vi "Dashboard Main.vi"() -> ()   [LabVIEW 2015]
uses:
  <vilib>/Utility/miscctls.llb/LVRowAndColumnTypeDef.ctl
  <vilib>/event_ctls.llb/eventvkey.ctl
  <vilib>/Rock Robotics/WPI/Dashboard/WPI_DashboardLogging Global.vi
  <vilib>/Rock Robotics/Network Tables/NT Read Numeric Array.vi
  <vilib>/Rock Robotics/Network Tables/NT Read Boolean.vi
  <vilib>/Rock Robotics/Network Tables/NT Write Boolean.vi
  <vilib>/Rock Robotics/Network Tables/NT Write Boolean Array.vi
  <vilib>/Rock Robotics/Network Tables/NT Write Numeric Array.vi
  <vilib>/Utility/config.llb/Write Key (String).vi
  <vilib>/Utility/config.llb/Write Key (I32).vi
  <vilib>/Utility/config.llb/NI_LVConfig.lvlib
panel:
  in  "TCP":refnum<k5>
  in  "Rec Mode":enum32{"Stop", "Record", "Playback"}(radio)
  in  "Vision":u16(ring)=1 items=["Camera Off", "USB Camera SW", "USB Camera HW", "IP Camera"]
  out "Camera IP":string
  out "Image Message":string="Timeout in Camera Communications"
  in  "Dashboard Tab":T1(tab)
  in  "Select Auto":string(combo)
  out "NT Connection":bool
  in  "Camera Settings":T2={"Frame Rate"=30, "Compression"=30, "Size"=1} {"Frame Rate" scale=1.0..30.0; "Size" items=["640x480", "320x240", "160x120"]}
  out "MotorChart R":cluster{"Numeric":dbl, "Numeric":dbl}(graph)
  out "MotorChart L":T3(graph)
  out "MotorSliders R":cluster{"MotorSlide1":dbl, "MotorSlide2":dbl} {"MotorSlide2" scale=-1.0..1.0 scale format="%#_2e"; "MotorSlide1" scale=-1.0..1.0 scale format="%#_2e"}
  out "MotorSliders L":T4 {"MotorSlide4 2" scale=0.0..14.0 scale format="%#_2e"; "MotorSlide2" scale=-1.0..1.0 scale format="%#_2e"; "MotorSlide1" scale=-1.0..1.0 scale format="%#_2e"}
  out "Gyro":dbl(knob) scale=0.0..360.0
  out "JS1 Z":dbl(slide) scale=-1.0..1.0 scale format="%#_2e"
  out "JS1 Graph":cluster{"X":dbl, "Y":dbl}[](graph)
  out "JS1 Buttons":T5
  out "JS2 Z":dbl(slide) scale=-1.0..1.0 scale format="%#_2e"
  out "JS2 Graph":cluster{"X":dbl, "Y":dbl}[](graph)
  out "JS2 Buttons":T5
  out "Mode":T6(ring)=enum."Auto Disabled"
  in  "DB Camera Config":bool
  out "fps":dbl format="%#.1g"
  out "Mbps":dbl format="%#.1g"
  out "Mbps LED":bool
  in  "DB/String 9":string
  in  "DB/String 8":string
  in  "DB/String 7":string
  in  "DB/String 6":string
  in  "DB/String 5":string
  in  "DB/String 4":string
  in  "DB/String 3":string
  in  "DB/String 2":string
  in  "DB/String 1":string
  in  "DB/String 0":string
  in  "DB/Slider 0":dbl(slide) scale=0.0..5.0
  in  "DB/Slider 1":dbl(slide) scale=0.0..5.0
  in  "DB/Slider 2":dbl(slide) scale=0.0..5.0
  in  "DB/Slider 3":dbl(slide) scale=0.0..5.0
  out "DB/LED 3":bool
  out "DB/LED 2":bool
  out "DB/LED 1":bool
  out "DB/LED 0":bool
  in  "DB/Button 3":bool
  in  "DB/Button 2":bool
  in  "DB/Button 1":bool
  in  "DB/Button 0":bool caption="New Name"
  in  "Rampart":bool
  in  "CL":dbl
  in  "Exposure Percentage":dbl
  in  "Brightness":dbl
  in  "Blue":cluster{"Low":dbl, "High":dbl}={"Low"=100.0, "High"=200.0}
  in  "Green":cluster{"Low":dbl, "High":dbl}={"Low"=100.0, "High"=230.0}
  in  "Red":cluster{"Low":dbl, "High":dbl}={"Low"=0.0, "High"=100.0}
  in  "Taking A Shot":bool
  in  "Position 4":bool
  in  "Position 3":bool
  in  "Position 2":bool
  in  "Position 1":bool
  out "Robot Aligned Straight":bool
  out "Ball In Position":bool
  in  "Test Slider":dbl(slide) scale=0.0..100.0 scale format="%#_3g"
  in  "On/Off":bool caption="Solenoid"
  in  "Test Name":u16(ring) items=["Select the test to run..."]
  in  "Test Tree":string(tree)
  in  "Motor":cluster{"Value":dbl, "Enable":bool} {"Value" scale=-1.0..1.0 scale format="%#_3g"}
  out "Progress":T7 {"Test Progress" scale=0.0..100.0}
  in  "Rev/Fwd":cluster{"Forward":bool, "Reverse":bool}
  in  "Test Ring":u16(ring) items=["Monochrome", "Color"]
  out "Cmd Status":string
  in  "Execute Command":bool
  in  "Command Params":string[][](table)
  in  "Command Selection":i32(listbox)
  in  "CheckList":i32(listbox)
  out "Tree":string(tree)
  out "Camera Image":T8(plugin-control)
  out "Background":bool
  # "Left"
  # "Front"
  # "Right"
  # "Battery"
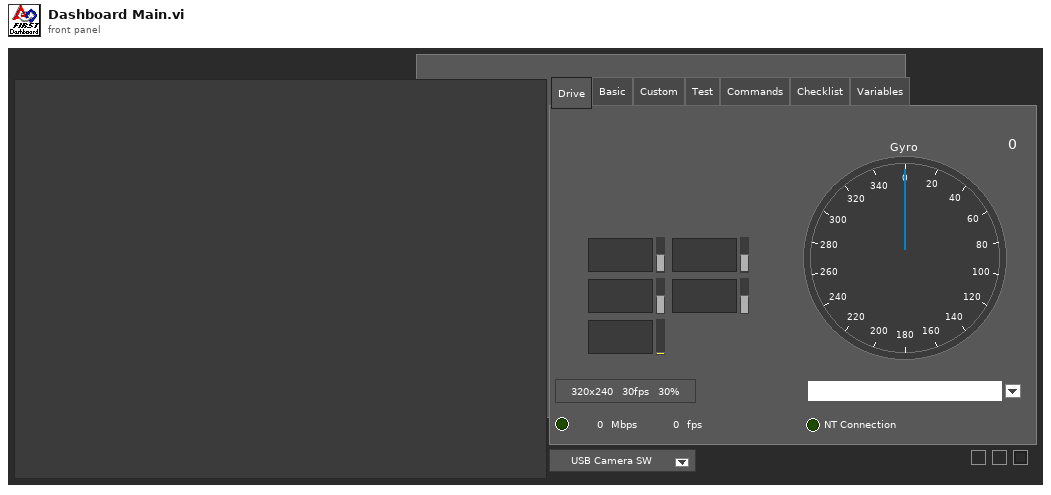
[diagram p1: front panel]
types:
  T1 = enum32{"Drive", "Basic", "Custom", "Test", "Commands", "Checklist", "Variables"}
  T2 = cluster{"Frame Rate":i32, "Compression":i32, "Size":u16}
  T3 = cluster{"Numeric":dbl, "Numeric":dbl, "Battery V":dbl}
  T4 = cluster{"MotorSlide1":dbl, "MotorSlide2":dbl, "MotorSlide4 2":dbl}
  T5 = cluster{bool, bool, bool, bool, bool, bool, bool, bool, bool, bool, bool, bool}
  T6 = enum8{"Tele-Op Disabled", "Tele-Op Enabled", "Auto Disabled", "Auto Enabled", "Test Disabled", "Test Enabled", "Disconnected", "No Code", "E-Stop"}
  T7 = cluster{"Test Progress":u8, "Test Progress Text":string}
  T8 = typedef "IMAQ Image.ctl" = refnum<image>
  T9 = cluster{"IDs":cluster{"RPC field ID":u16, "Unique ID":u16}, "String":string}
  T10 = enum32{"Drive", "Basic", "Custom", "Test", "Checklist", "Variables"}
  T11 = typedef "Image Type" = u32
  T12 = cluster{"Camera Image":refnum<vi>, "Dashboard Tab":refnum<vi>, "Background":refnum<vi>, "Vision":refnum<vi>, "Rec Mode":refnum<vi>, "Test Slider":refnum<vi>, "On/Off ":refnum<vi>, "Test Ring":refnum<vi>, "Rev/Fwd":refnum<vi>, "Test Name":refnum<vi>, "Motor":refnum<vi>, "Progress":refnum<vi>, "CheckList":refnum<vi>, "Tree":refnum<vi>, "Test Tree":refnum<vi>, "Command Params":refnum<vi>, "Command Selection":refnum<vi>, "Execute Command":refnum<vi>, "Cmd Status":refnum<vi>}
  T13 = cluster{"Error Strings":string, "Disable Counts":cluster{u16, u16}, "Rail Faults":cluster{u16, u16, u16}, "Robot IP":string, "DB Mode":u8, "Event Info":cluster{"Name":string, "Type":u8, "Number":u16, "Replay":u8}, "Camera Addr":string}
  T14 = cluster{"Storage":cluster{"Disk Free":u64, "RAM Block":u32, "RAM free":u32}, "CPU Utilization":cluster{"CPU % ISR":sgl, "CPU % Time Crit":sgl, "CPU % Timed Str":sgl, "CPU % High":sgl, "CPU % Above":sgl, "CPU % Normal":sgl, "CPU % Low":sgl}, "CAN":cluster{"% Bus Utilization":sgl, "Bus Off Cnt":u32, "TX_FIFO Full Cnt":u32, "Receive Error Cnt":u8, "Transmit Error Cnt":u8}, "HID":cluster{"HID Outputs":u32, "Rumble Low":u16, "Rumble High":u16}[]}
  T15 = cluster{"Status bits":cluster{"Test Mode":bool, "Autonomous":bool, "Enabled":bool, "Code Start":bool, "Brownout":bool, "Reserved 2":bool, "Reserved 3":bool, "E-Stop":bool}, "Code Trace":cluster{"Disabled":bool, "TeleOp":bool, "Auto":bool, "Test":bool}, "Controller Type":enum16{"unknown", "cRIO", "roboRio"}, "Code?":enum16{"unknown", "noCode", "code"}, "Battery V":dbl}
  T16 = cluster{"Control Bits":cluster{"TestMode":bool, "Autonomous":bool, "Enabled":bool, "FMS Present":bool, bool, bool, bool, "E-Stop":bool}, "Team Station ":u8, "Countdown":sgl, "Joystick Values":cluster{"Axes":dbl[], "Buttons":bool[], "POVs":i16[]}[]}
  T17 = cluster{"Axes":dbl[], "Buttons":bool[], "POVs":i16[]}[]
  T18 = cluster{"Axes":dbl[], "Buttons":bool[], "POVs":i16[]}
  T19 = cluster{"Buttons[0]":bool, "Buttons[1]":bool, "Buttons[2]":bool, "Buttons[3]":bool, "Buttons[4]":bool, "Buttons[5]":bool, "Buttons[6]":bool, "Buttons[7]":bool, "Buttons[8]":bool, "Buttons[9]":bool, "Buttons[10]":bool, "Buttons[11]":bool}
  T20 = typedef "NI_LVConfig.lvlib/Config Data RefNum.ctl" = refnum<k1>
  T21 = cluster{"Operation":enum16{"Update", "Clear"}, "Color Box":u32}[]
  T22 = typedef "eventvkey.ctl" = enum16{"ASCII", "Enter", "Return", "Shift", "Ctrl", "Alt", "Cmd", "Opt", "Caps", "NumLock", "Clear", "Break", "Up", "Down", "Left", "Right", "Insert", "Delete", "Home", "End", "PageUp", "PageDown", "Escape", "Help", "Pause", "ScrollLock", "F1", "F2", "F3", "F4", "F5", "F6", "F7", "F8", "F9", "F10", "F11", "F12", "F13", "F14", "F15", "F16", "F17", "F18", "F19", "F20", "F21", "F22", "F23", "F24", "Play", "VolumeUp", "VolumeDown", "Mute", "Two Byte Char"}
  T23 = cluster{"Image Size":bool, "Image Type":bool, "Pixel Value":bool, "ROI Information":bool, "Zoom Factor":bool}
  T24 = enum8{"Enabled", "Disabled", "Disabled and Grayed Out"}
  T25 = cluster{"Operation":enum16{"Update", "Clear"}, "Color Box":u32}
  T26 = typedef "LVRowAndColumnTypeDef.ctl" = cluster{"Row":i32, "Column":i32}
  T27 = cluster{"Shift":bool, "Ctrl":bool, "Alt":bool, "Cmd":bool, "Opt":bool}
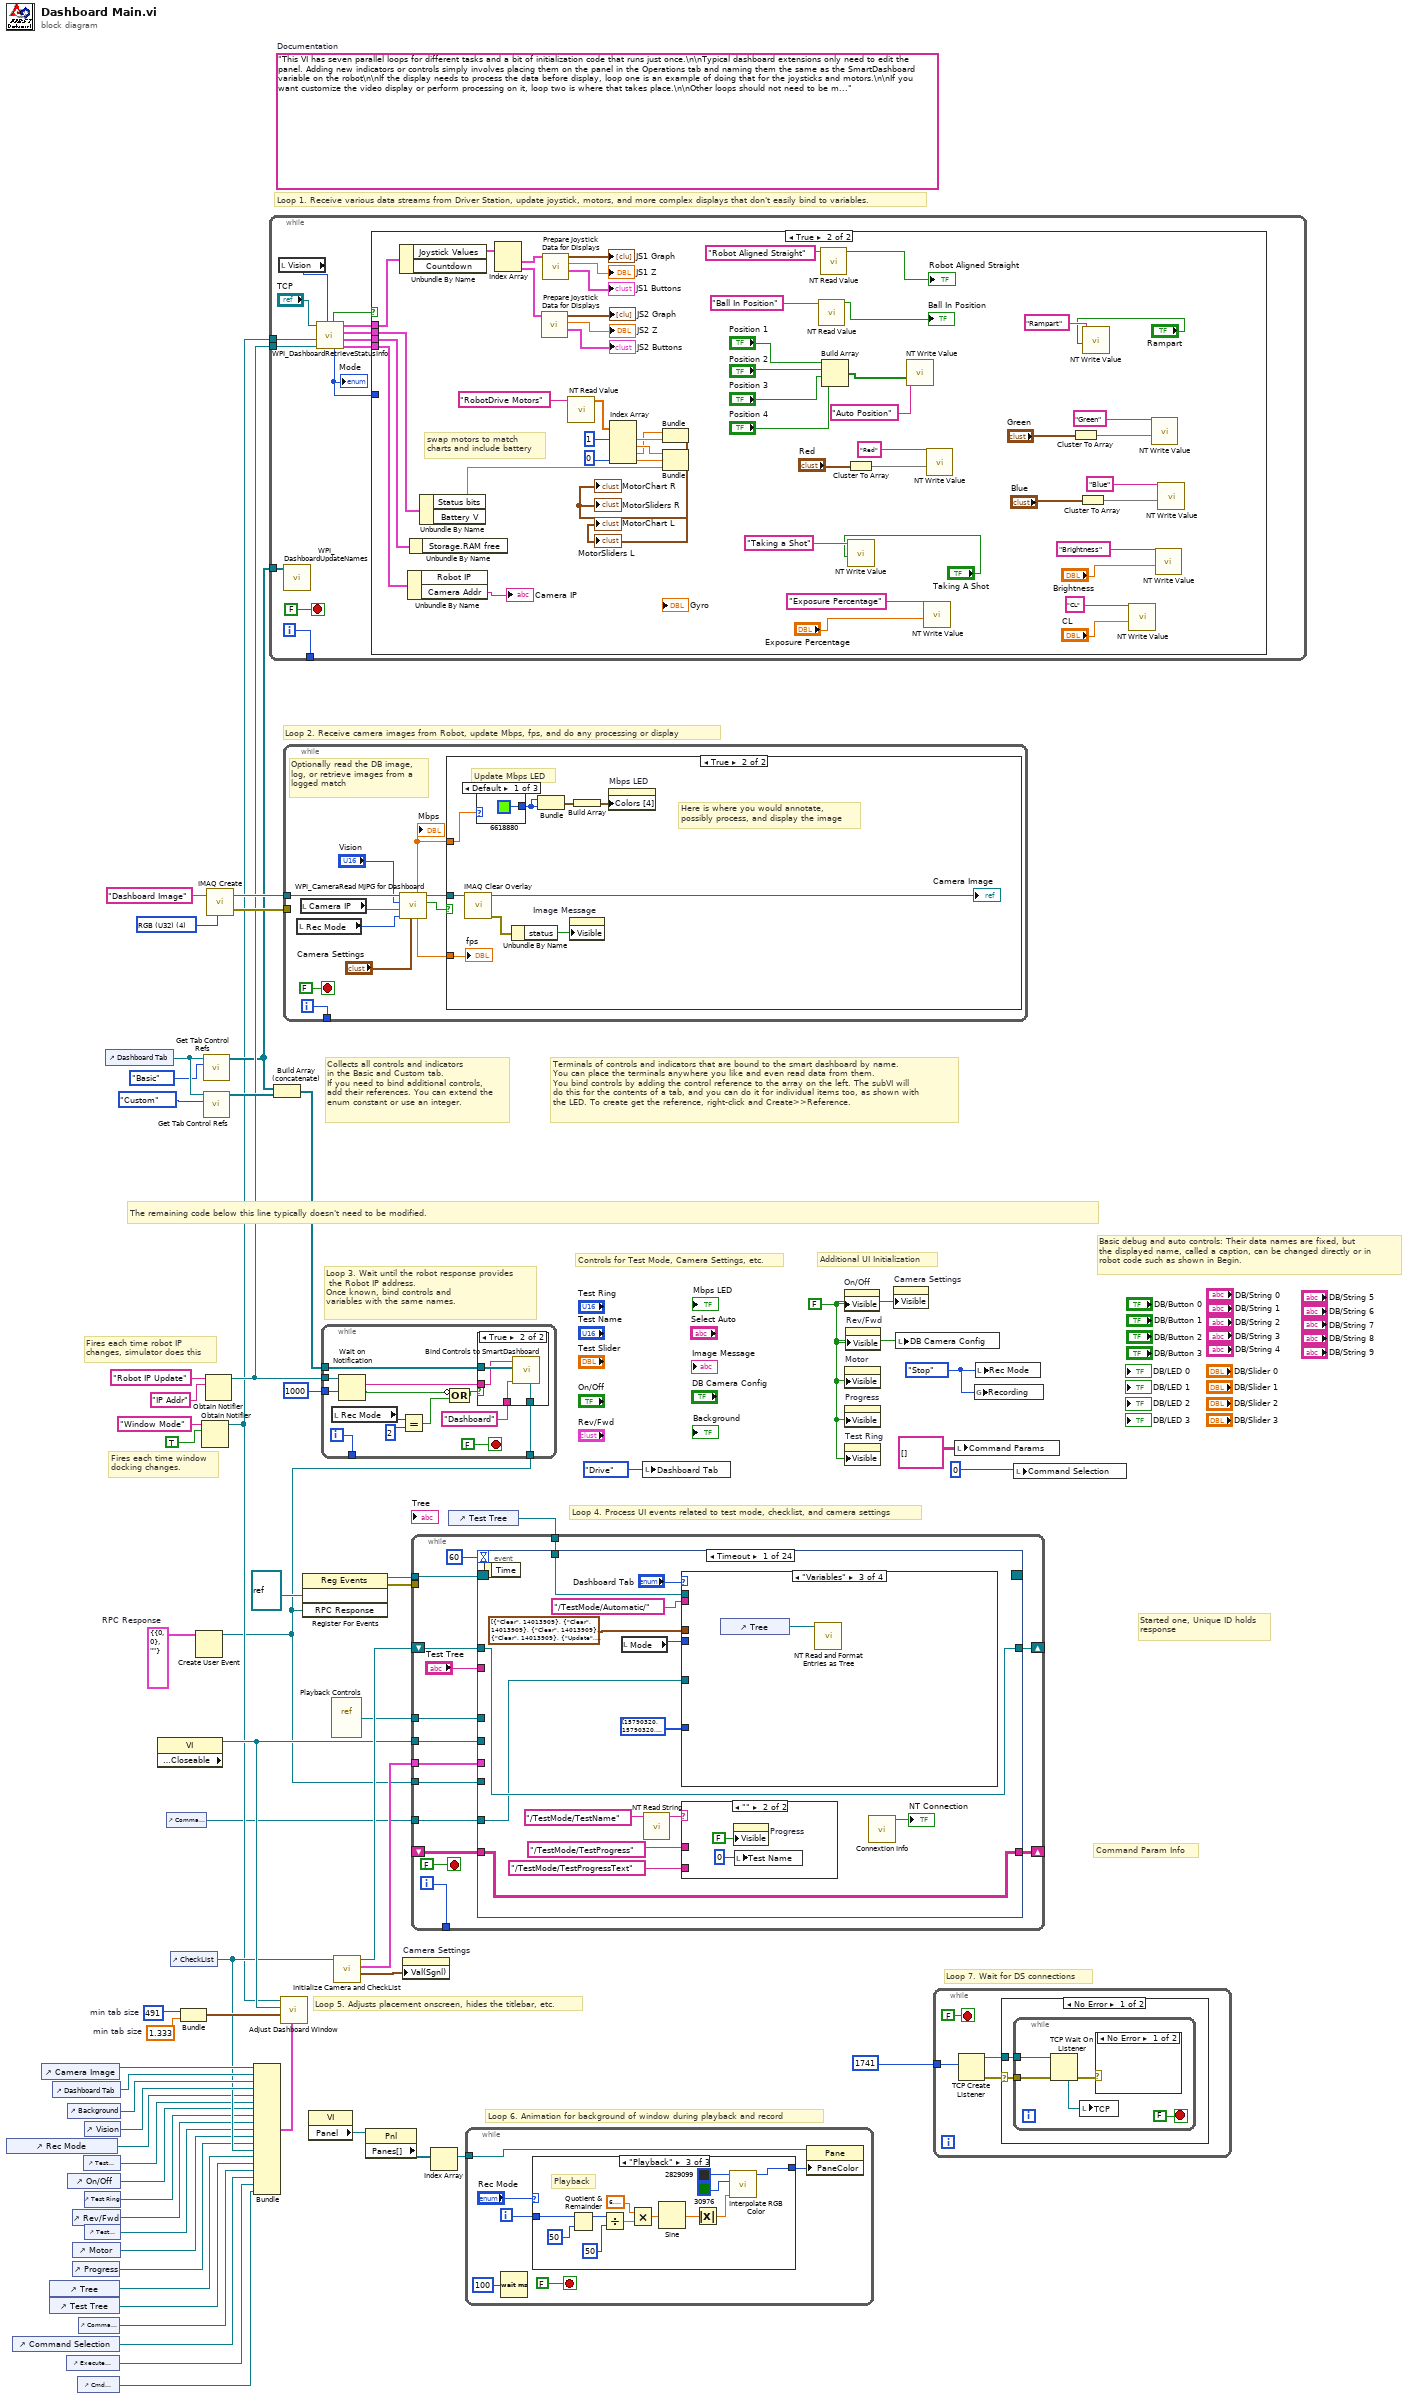
[diagram p0: block diagram]
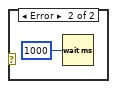
[diagram p2: hidden frame]
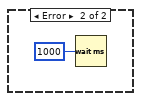
[diagram p3: hidden frame]
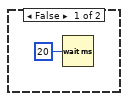
[diagram p4: hidden frame]
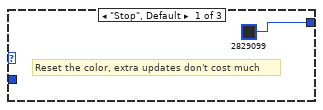
[diagram p5: hidden frame]
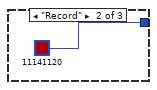
[diagram p6: hidden frame]
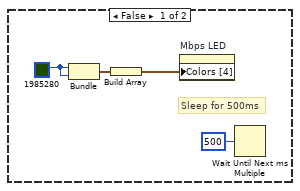
[diagram p8: hidden frame]
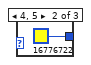
[diagram p9: hidden frame]
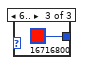
[diagram p10: hidden frame]
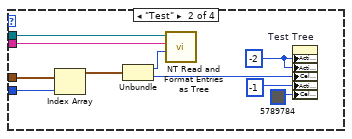
[diagram p12: hidden frame]
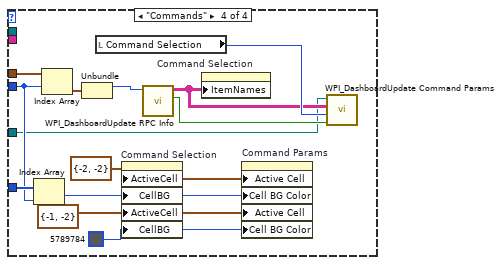
[diagram p13: hidden frame]
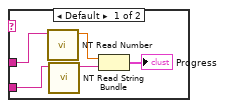
[diagram p14: hidden frame]
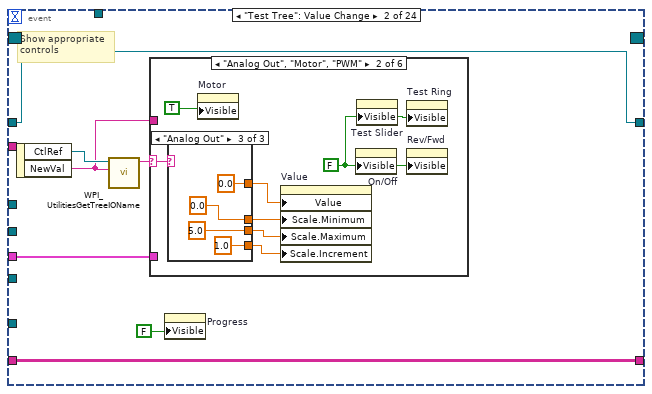
[diagram p15: hidden frame]
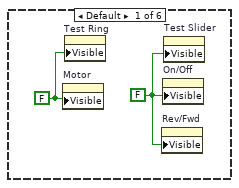
[diagram p16: hidden frame]
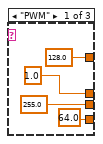
[diagram p17: hidden frame]
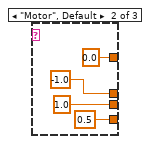
[diagram p18: hidden frame]
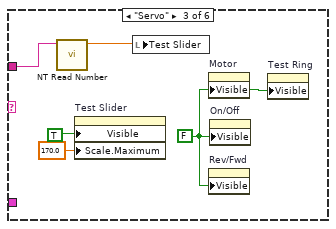
[diagram p19: hidden frame]
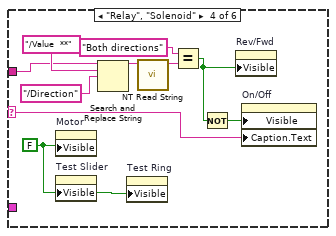
[diagram p20: hidden frame]
diagram:
  w7 = T9 {"IDs"={"RPC field ID"=0, "Unique ID"=0}, "String"=""}  # RPC Response
  w33 = 491  # min tab size
  w32 = 1.333  # min tab size
  w41 = enum32{"Stop", "Record", "Playback"}."Stop" ("Rec Mode")
  w15 = FALSE ("Visible")
  (unwired) "This VI has seven parallel loops for different tasks and a bit of initialization code that runs just once.\n\nTypical dashboard extensions only need to edit the panel. Adding new indicators or controls simply involves placing them on the panel in the Operations tab and naming them the same as the SmartDashboard variable on the robot\n\nIf the display needs to process the data before display, loop one is an example of doing that for the joysticks and motors.\n\nIf you want customize the video display or perform processing on it, loop two is where that takes place.\n\nOther loops should not need to be modified. They are pretty standard, and document the task they perform."  # Documentation
  w61 = T11 4 items=["Grayscale (U8)", "Grayscale (I16)", "Grayscale (SGL)", "Complex (CSG)", "RGB (U32)", "HSL (U32)", "RGB (U64)"] ("Image Type")
  # "Command Param Info"
  # "Started one, Unique ID holds\nresponse"
  # "Loop 7. Wait for DS connections"
  # "Basic debug and auto controls: Their data names are fixed, but\nthe displayed name, called a caption, can be changed directly or in\nrobot code such as shown in Begin."
  # "Controls for Test Mode, Camera Settings, etc."
  # "Additional UI Initialization"
  # "Loop 6. Animation for background of window during playback and record"
  # "Fires each time robot IP\nchanges, simulator does this"
  # "Fires each time window\ndocking changes."
  # "Collects all controls and indicators\nin the Basic and Custom tab.\nIf you need to bind additional controls,\nadd their references. You can extend the\nenum constant or use an integer."
  # "The remaining code below this line typically doesn't need to be modified."
  # "Loop 4. Process UI events related to test mode, checklist, and camera settings"
  # "Terminals of controls and indicators that are bound to the smart dashboard by name.\nYou can place the terminals anywhere you like and even read data from them.\nYou bind controls by adding the control reference to the array on the left. The subVI will\ndo this for the contents of a tab, and you can do it for individual items too, as shown with\nthe LED. To create get the reference, right-click and Create>>Reference."
  # "Loop 3. Wait until the robot response provides\n the Robot IP address.\nOnce known, bind controls and\nvariables with the same names."
  # "Loop 5. Adjusts placement onscreen, hides the titlebar, etc."
  # "Loop 1. Receive various data streams from Driver Station, update joystick, motors, and more complex displays that don't easily bind to variables."
  # "Loop 2. Receive camera images from Robot, update Mbps, fps, and do any processing or display"
  n1 = control-ref of="Rec Mode"() -> (w21:refnum<vi>)
  n2 = control-ref of="Command Selection"() -> (w6:refnum<vi>)
  n3 = control-ref of="Camera Image"() -> (w36:refnum<vi>)
  n4 = control-ref of="Tree"() -> (w25:refnum<vi>)
  n5 = control-ref of="Test Tree"() -> (w24:refnum<vi>)
  n6 = control-ref of="Dashboard Tab"() -> (w35:refnum<vi>)
  n7 = control-ref of="Execute Command"() -> (w8:refnum<vi>)
  n8 = control-ref of="Background"() -> (w30:refnum<vi>)
  n9 = control-ref of="On/Off"() -> (w19:refnum<vi>)
  n10 = control-ref of="Progress"() -> (w16:refnum<vi>)
  n11 = control-ref of="Rev/Fwd"() -> (w17:refnum<vi>)
  n12 = control-ref of="Motor"() -> (w22:refnum<vi>)
  n13 = control-ref of="Cmd Status"() -> (w2:refnum<vi>)
  n14 = control-ref of="Command Params"() -> (w9:refnum<vi>)
  n15 = control-ref of="Test Slider"() -> (w20:refnum<vi>)
  n16 = control-ref of="Vision"() -> (w34:refnum<vi>)
  n17 = control-ref of="Test Ring"() -> (w18:refnum<vi>)
  n18 = control-ref of="Test Name"() -> (w23:refnum<vi>)
  n19 = control-ref of="Dashboard Tab"() -> (w39:refnum<vi>)
  n20 = property class="VI" props=["Front Panel.Closeable"]() -> (reference out=w40:refnum<vi>)  [unwired: 2 in, 2 out]
  n21 = control-ref of="Command Params"() -> (w1:refnum<vi>)
  n22 = control-ref of="CheckList"() -> (w26:refnum<vi>)
  n23 = Bundle("min tab size"=w33, "min tab size"=w32) -> (w31:cluster{"min tab size":i32, "min tab size":dbl})  [unwired: 1 in]
  n24 = Create User Event(user event datatype=w7) -> (user event=w3:refnum<user-event>)  [unwired: 1 in, 1 out]
  n25 = Obtain Notifier(name (unnamed)="Window Mode", notification data type=TRUE) -> (notifier out=w12:refnum<notifier>)  [unwired: 2 in, 2 out]
  n26 = call <vilib>:"Get Tab Control Refs.vi"("Page Index"=T10."Basic" ("Dashboard Tab"), "TabControl in"=w39) -> ("ControlsOnPage"=w13:refnum<vi>[])  [unwired: 9 in]
  n27 = call <vilib>:"Get Tab Control Refs.vi"("Page Index"=T10."Custom" ("Dashboard Tab"), "TabControl in"=w39) -> ("ControlsOnPage"=w38:refnum<vi>[])  [unwired: 9 in]
  n28 = Obtain Notifier(name (unnamed)="Robot IP Update", notification data type="IP Addr" ("name (unnamed)")) -> (notifier out=w14:refnum<notifier>)  [unwired: 2 in, 2 out]
  n29 = call "IMAQ Create"("Image Name"="Dashboard Image", "Image Type"=w61) -> ("New Image"=w59:T8, "error out"=w58:errorcluster)  [unwired: 2 in, 1 out]
  n30 = Bundle("Camera Image"=w36, "Dashboard Tab"=w35, "Background"=w30, "Vision"=w34, "Rec Mode"=w21, "Test Slider"=w20, "On/Off"=w19, "Test Ring"=w18, "Rev/Fwd"=w17, "Test Name"=w23, "Motor"=w22, "Progress"=w16, "CheckList"=w26, "Tree"=w25, "Test Tree"=w24, "Command Params"=w9, "Command Selection"=w6, "Execute Command"=w8, "Cmd Status"=w2) -> (w27:T12)  [unwired: 1 in]
  n31 = while {
    tunnel: [w73] -> _
    tunnel: w14 -> [w67]
    tunnel: w13 -> [w66]
    tunnel: w12 -> [w62]
    i -> [w73]
    stop <- FALSE stop-if-true
    n32 = local read "Vision"() -> (w64:u16)
    n33 = call <vilib>:"WPI_DashboardUpdateNames.vi"("Controls on Tab"=w66) -> ()  [unwired: 11 in]
    n34 = call <vilib>:"WPI_DashboardRetrieveStatusInfo.vi"("Vision"=w64, "Binding Refnum"=w67, "Window Mode Notifier"=w62, "TCP Cnx"="TCP") -> ("Power and Errors"=w68:T13, "Robot Metrics"=w71:T14, "Status Info"=w72:T15, "Control Info"=w69:T16, "Robot Mode"=w65:T6, "Process?"=w70:bool)  [unwired: 2 in]
    "Mode" <- w65
    n35 = case shown="True" w70 {
      tunnel: w72 -> [_ w129]
      tunnel: w71 -> [_ w128]
      tunnel: w69 -> [_ w127]
      tunnel: w68 -> [_ w126]
      tunnel: w65 -> [_ _]
      frame False {
        n36 = Wait (ms)(milliseconds to wait=u32 20) -> ()  [unwired: 1 out]
      }
      frame True {
        # "swap motors to match\ncharts and include battery"
        n37 = Unbundle By Name(w127) -> ("Joystick Values"=w116:T17)  [unwired: 1 out]
        n38 = Unbundle By Name(w126) -> ("Camera Addr"=→"Camera IP":string)  [unwired: 1 out]
        n39 = Unbundle By Name(w128) -> ()  [unwired: 1 out]
        n40 = Unbundle By Name(w129) -> ("Battery V"=w117:dbl)  [unwired: 1 out]
        n41 = Index Array(array=w116) -> (element #1=w115:T18, element #2=w110:T18)  [unwired: 2 in]
        n42 = call "Prepare Joystick Data for Displays.vi"("Joystick Values"=w110) -> ("Buttons"=→"JS2 Buttons":T19, "Z Axis"=→"JS2 Z":dbl, "Cartesian Data"=→"JS2 Graph":cluster{"X axis":dbl, "X axis":dbl}[])  [unwired: 8 in]
        n43 = call "Prepare Joystick Data for Displays.vi"("Joystick Values"=w115) -> ("Buttons"=→"JS1 Buttons":T19, "Z Axis"=→"JS1 Z":dbl, "Cartesian Data"=→"JS1 Graph":cluster{"X axis":dbl, "X axis":dbl}[])  [unwired: 8 in]
        n44 = call-poly <vilib>:"NT Read Value.vi"("Name"="RobotDrive Motors") -> ("Numeric Array"=w105:dbl[])  [unwired: 9 in, 1 out]
        n45 = Index Array(array=w105, index #1=1, index #4=0) -> (element #1=w121:dbl, element #2=w122:dbl, element #3=w120:dbl, element #4=w125:dbl)  [unwired: 2 in]
        n46 = Bundle("Numeric"=w120, "Numeric"=w121) -> (→"MotorChart R" →"MotorSliders R":cluster{"Numeric":dbl, "Numeric":dbl})  [unwired: 1 in]
        n47 = Bundle("Numeric"=w122, "Numeric"=w125, "Battery V"=w117) -> (→"MotorChart L" →"MotorSliders L":T3)  [unwired: 1 in]
        n48 = call-poly <vilib>:"NT Read Value.vi"("Name"="Ball In Position") -> ("Boolean"=→"Ball In Position":bool)  [unwired: 9 in, 1 out]
        n49 = call-poly <vilib>:"NT Read Value.vi"("Name"="Robot Aligned Straight") -> ("Boolean"=→"Robot Aligned Straight":bool)  [unwired: 9 in, 1 out]
        n50 = Build Array("Position 1", "Position 2", "Position 3", "Position 4") -> (w93:bool[])
        n51 = Cluster To Array(cluster="Red") -> (array=w89:dbl[])
        n52 = call-poly <vilib>:"NT Write Value.vi"("Boolean"="Taking A Shot", "Name"="Taking a Shot") -> ()  [unwired: 9 in, 1 out]
        n53 = call-poly <vilib>:"NT Write Value.vi"("Boolean Array"=w93, "Name"="Auto Position") -> ()  [unwired: 9 in, 1 out]
        n54 = call-poly <vilib>:"NT Write Value.vi"("Numeric"="Exposure Percentage", "Name"="Exposure Percentage") -> ()  [unwired: 9 in, 1 out]
        n55 = call-poly <vilib>:"NT Write Value.vi"("Numeric Array"=w89, "Name"="Red") -> ()  [unwired: 9 in, 1 out]
        n56 = Cluster To Array(cluster="Green") -> (array=w88:dbl[])
        n57 = Cluster To Array(cluster="Blue") -> (array=w85:dbl[])
        n58 = call-poly <vilib>:"NT Write Value.vi"("Boolean"="Rampart", "Name"="Rampart") -> ()  [unwired: 9 in, 1 out]
        n59 = call-poly <vilib>:"NT Write Value.vi"("Numeric"="CL", "Name"="CL") -> ()  [unwired: 9 in, 1 out]
        n60 = call-poly <vilib>:"NT Write Value.vi"("Numeric Array"=w88, "Name"="Green") -> ()  [unwired: 9 in, 1 out]
        n61 = call-poly <vilib>:"NT Write Value.vi"("Numeric"="Brightness", "Name"="Brightness") -> ()  [unwired: 9 in, 1 out]
        n62 = call-poly <vilib>:"NT Write Value.vi"("Numeric Array"=w85, "Name"="Blue") -> ()  [unwired: 9 in, 1 out]
      }
    }
  }
  n63 = Build Array (concatenate)(w13, w38) -> (w37:refnum<vi>[])
  n64 = call "Adjust Dashboard Window.vi"("Sizing Refnums"=w27, "Size Constraints"=w31, "VI"=w40, "WIn Mode"=w12) -> ()  [unwired: 8 in]
  n65 = while {
    tunnel: w59 -> [w138]
    tunnel: w58 -> [_]
    tunnel: [w139] -> _
    i -> [w139]
    stop <- FALSE stop-if-true
    # "Optionally read the DB image,\nlog, or retrieve images from a\nlogged match"
    n66 = local read "Rec Mode"() -> (w133:enum32{"Stop", "Record", "Playback"})
    n67 = local read "Camera IP"() -> (w131:string)
    n68 = call <vilib>:"WPI_CameraRead MJPG for Dashboard.vi"("Camera Settings"="Camera Settings", "Rec Mode"=w133, "Camera IP"=w131, "Camera Mode"="Vision", "Refnum in"=w138) -> ("Active"=w136:bool, "Refnum out"=w137:T8, "FPS"=w135:dbl, "Bandwidth (Mbps)"=w130:dbl)  [unwired: 3 in]
    "Mbps" <- w130
    n69 = case shown="True" w136 {
      tunnel: w137 -> [_ w148]
      tunnel: w130 -> [_ w147]
      tunnel: w135 -> [_ w145]
      frame False {
        w141 = u32 1985280 ("Color Box")
        # "Sleep for 500ms"
        n70 = Bundle("Color Box"=w141, "Color Box"=w141) -> (w143:cluster{"Color Box":u32, "Color Box":u32})  [unwired: 1 out]
        n71 = Build Array(w143) -> (w142:cluster{"Color Box":u32, "Color Box":u32}[])
        n72 = property on="Mbps LED" class="Bool (strict)"("Colors [4]"=w142) -> ()  [unwired: 2 in, 2 out]
        n73 = Wait Until Next ms Multiple(millisecond multiple=u32 500) -> ()  [unwired: 1 out]
      }
      frame True {
        # "Here is where you would annotate,\npossibly process, and display the image"
        # "Update Mbps LED"
        n74 = call "IMAQ Clear Overlay"("Image"=w148) -> ("error out"=w152:errorcluster, "Image Out"=→"Camera Image":T8)  [unwired: 2 in, 7 out]
        n75 = case shown="Default" w147 {
          tunnel: [u32 6618880 ("Color Box") u32 16776722 ("Color Box") u32 16716800 ("Color Box")] -> w149
          frame Default {
          }
          frame 4, 5 {
          }
          frame 6.. {
          }
        }
        n76 = Unbundle By Name(w152) -> ("status"=w153:bool)
        n77 = Bundle("Color Box"=w149, "Color Box"=w149) -> (w151:cluster{"Color Box":u32, "Color Box":u32})  [unwired: 1 out]
        n78 = property on="Image Message" class="Str"("Visible"=w153) -> ()  [unwired: 2 in, 2 out]
        n79 = Build Array(w151) -> (w150:cluster{"Color Box":u32, "Color Box":u32}[])
        n80 = property on="Mbps LED" class="Bool (strict)"("Colors [4]"=w150) -> ()  [unwired: 2 in, 2 out]
        "fps" <- w145
      }
    }
  }
  n81 = register-events(refnum<vi> refnum, w3) -> (reference out=w45:refnum<event-registration>, error out=w44:errorcluster)  [unwired: 2 in]
  n82 = property class="VI"() -> ("Panel"=w48:refnum<vi>)  [unwired: 2 in, 2 out]
  n83 = while {
    tunnel: w37 -> [w169]
    tunnel: w14 -> [w167]
    tunnel: [w165] -> _
    tunnel: u32 1000 ("milliseconds to wait") -> [w164]
    tunnel: w3 -> [w157]
    i -> [w165]
    stop <- FALSE stop-if-true
    n84 = local read "Rec Mode"() -> (w160:enum32{"Stop", "Record", "Playback"})
    n85 = Wait on Notification(notifier=w167, timeout in ms (-1)=w164) -> (notification=w166:string, timed out?=w162:bool)  [unwired: 2 in, 2 out]
    n86 = Equal?(x=w160, y=u16 2 ("Rec Mode")) -> (x = y?=w161:bool)
    n87 = Compound Arithmetic op=OR(invert w162, w161) -> (w163:bool)
    n88 = case shown="True" w163 {
      tunnel: w169 -> [_ w173]
      tunnel: w166 -> [_ w172]
      tunnel: "Dashboard" -> [_ w171]
      tunnel: w157 -> [_ w170]
      frame False {
      }
      frame True {
        n89 = call <vilib>:"Bind Controls to SmartDashboard.vi"("RPC ref"=w170, "Client Name"=w171, "Bound Control Refs"=w173, "Server IP Address"=w172) -> ()  [unwired: 8 in]
      }
    }
  }
  n90 = vi-ref "Playback Controls.vi"() -> (w46:refnum<vi>)
  n91 = call "Initialize Camera and CheckList.vi"("ListBox in"=w26) -> ("Cluster"=w52:cluster{"value":i32, "value":i32, "index":i32}, "Array"=w53:cluster{string[]}[], "File Refnum"=w51:T20)  [unwired: 8 in]
  n92 = property class="Pnl"(reference=w48) -> ("Panes[]"=w49:refnum<vi>[])  [unwired: 1 in, 2 out]
  n93 = property on="Camera Settings" class="Clust (strict)"("Val(Sgnl)"=w52) -> ()  [unwired: 2 in, 2 out]
  n94 = Index Array(array=w49) -> (element=w47:refnum<vi>)  [unwired: 1 in]
  n95 = control-ref of="Test Tree"() -> (w50:refnum<vi>)
  n96 = while {
    tunnel: w53 -> [w185]
    shift-right: [w184] -> _
    shift-left: w51 -> [w183]
    tunnel: [w182] -> _
    tunnel: w50 -> [w181]
    tunnel: w46 -> [w180]
    tunnel: w45 -> [w179]
    tunnel: w44 -> [_]
    tunnel: w40 -> [w178]
    tunnel: w3 -> [w177]
    tunnel: w1 -> [w176]
    shift-right: [w175] -> _
    shift-left: _ -> [w174]
    i -> [w182]
    stop <- FALSE stop-if-true
    n97 = event shown="[0] Timeout" {
      selector: w179 -> [_ _ _ _ _ _ _ _ _ _ _ _ _ _ _ _ _ _ _ _ _ _ _ _]
      dyn-events: [_ _ _ _ _ _ _ _ _ _ _ _ _ _ _ _ _ _ w494 _ _ _ _ _] -> _
      timeout: u32 60 ("milliseconds to wait") -> [_ _ _ _ _ _ _ _ _ _ _ _ _ _ _ _ _ _ _ _ _ _ _ _]
      tunnel: w181 -> [w198 _ _ _ _ _ _ _ _ _ _ _ _ _ _ _ _ _ _ _ _ _ _ _]
      tunnel: "Test Tree" -> [_ _ _ _ _ _ _ _ _ _ _ _ _ w457 w466 w469 w474 w483 _ _ _ _ _ _]
      tunnel: w185 -> [_ w236 _ _ _ _ _ _ _ _ _ w419 w450 _ _ _ _ _ _ _ _ _ _ _]
      tunnel: [w195 w235 w339 w345 w355 w359 w365 w377 w385 w391 w404 w418 w443 w456 w464 w468 w473 w482 w496 w512 w514 w522 w533 w538] -> w184
      tunnel: w183 -> [w195 w235 w339 w345 w355 w359 w365 w377 w385 w391 w404 w417 w443 w456 w464 w468 w473 w482 w496 w512 w514 w522 w533 w538]
      tunnel: w180 -> [_ _ _ _ _ _ _ _ _ _ _ _ _ _ _ _ _ _ w497 _ w517 _ _ _]
      tunnel: w178 -> [_ _ _ _ _ _ _ _ _ _ _ _ _ _ _ _ _ _ w492 _ _ _ _ _]
      tunnel: w177 -> [_ _ _ _ _ _ _ _ _ _ _ _ _ _ _ _ _ _ w488 _ _ _ _ _]
      tunnel: w176 -> [w190 _ _ _ _ _ w363 _ _ _ _ _ _ _ _ _ _ _ _ _ _ _ _ _]
      tunnel: [w189 w234 w338 w344 w354 w360 w361 w371 w382 w390 w403 w416 w442 w455 w463 w467 w472 w481 w487 w510 w513 w518 w526 w539] -> w175
      tunnel: w174 -> [w189 w234 w338 w344 w354 w360 w361 _ _ w390 w403 w416 w442 w455 w463 w467 w472 w481 w487 w510 w513 w518 w526 w539]
      event Timeout {
        n98 = event-data() -> ()  [unwired: 1 in, 1 out]
        n99 = local read "Mode"() -> (w192:T6)
        n100 = call <vilib>:"NT Read String.vi"("Name"="/TestMode/TestName") -> ("String"=w201:string)  [unwired: 9 in, 1 out]
        n101 = case shown="\"Variables\"" "Dashboard Tab" {
          tunnel: w198 -> [_ w212 _ _]
          tunnel: "/TestMode/Automatic/" ("Name Pattern") -> [_ w211 _ _]
          tunnel: T21 [{"Operation"=enum."Clear", "Color Box"=14013909}, {"Operation"=enum."Clear", "Color Box"=14013909}, {"Operation"=enum."Clear", "Color Box"=14013909}, {"Operation"=enum."Clear", "Color Box"=14013909}, {"Operation"=enum."Update", "Color Box"=14013909}, {"Operation"=enum."Update", "Color Box"=16777215}, {"Operation"=enum."Clear", "Color Box"=14013909}, {"Operation"=enum."Clear", "Color Box"=14013909}, {"Operation"=enum."Clear", "Color Box"=14013909}] -> [_ w204 _ w221]
          tunnel: w192 -> [_ w203 _ w220]
          tunnel: u32[] [15790320, 15790320, 15790320, 15790320, 16777215, 16777215, 15790320, 15790320, 15790320] -> [_ _ _ w226]
          tunnel: w190 -> [_ _ _ w214]
          frame "Custom", Default {
          }
          frame "Test" {
            w210 = -2 ("Active Item:Row Number")
            n102 = Index Array(array=w204, index=w203) -> (element=w205:T25)
            n103 = Unbundle(w205) -> ("Operation"=w206:enum16{"Update", "Clear"}, "Color Box"=w207:u32)
            n104 = call <vilib>:"NT Read and Format Entries as Tree.vi"("Operation"=w206, "Name Pattern"=w211, "Tree Refnum"=w212) -> ()  [unwired: 7 in, 2 out]
            n105 = property on="Test Tree" class="Tree (strict)"("Active Item Row Number"=w210, "ActiveColNum"=w210, "CellBG"=w207, "Active Item Row Number"=-1 ("Active Item:Row Number"), "CellBG"=u32 5789784 ("Color Box")) -> ()  [unwired: 2 in, 2 out]
          }
          frame "Variables" {
            n106 = control-ref of="Tree"() -> (w213:refnum<vi>)
            n107 = call <vilib>:"NT Read and Format Entries as Tree.vi"("Tree Refnum"=w213) -> ()  [unwired: 9 in, 2 out]
          }
          frame "Commands" {
            w222 = u32 5789784 ("Color Box")
            w223 = T26 {"Row"=-1, "Column"=-2} ("Active Cell:Active Cell")
            w225 = T26 {"Row"=-2, "Column"=-2} ("Active Cell:Active Cell")
            n108 = Index Array(array=w226, index=w220) -> (element=w224:u32)
            n109 = Index Array(array=w221, index=w220) -> (element=w219:T25)
            n110 = Unbundle(w219) -> ("Operation"=w218:enum16{"Update", "Clear"})  [unwired: 1 out]
            n111 = local read "Command Selection"() -> (w217:i32)
            n112 = property on="Command Selection" class="MCListbox (strict)"("ActiveCell"=w225, "CellBG"=w224, "ActiveCell"=w223, "CellBG"=w222) -> ()  [unwired: 2 in, 2 out]
            n113 = call <vilib>:"WPI_DashboardUpdate RPC Info.vi"("Operation"=w218) -> ("update"=w216:bool, "commands"=w215:string[][])  [unwired: 9 in]
            n114 = property on="Command Selection" class="MCListbox (strict)"("ItemNames"=w215) -> ()  [unwired: 2 in, 2 out]
            n115 = property on="Command Params" class="Tbl (strict)"("Active Cell"=w225, "Cell BG Color"=w224, "Active Cell"=w223, "Cell BG Color"=w222) -> ()  [unwired: 2 in, 2 out]
            n116 = call <vilib>:"WPI_DashboardUpdate Command Params.vi"("Update"=w216, "NewVal"=w217, "Commands"=w215, "Param Tbl"=w214) -> ()  [unwired: 7 in, 1 out]
          }
        }
        n117 = case shown="\"\"" w201 {
          tunnel: "/TestMode/TestProgress" ("Name") -> [w228 _]
          tunnel: "/TestMode/TestProgressText" ("Name") -> [w227 _]
          frame Default {
            n118 = call <vilib>:"NT Read Number.vi"("Name"=w228) -> ("Numeric"=w229:dbl)  [unwired: 9 in, 1 out]
            n119 = call <vilib>:"NT Read String.vi"("Name"=w227) -> ("String"=w230:string)  [unwired: 9 in, 1 out]
            n120 = Bundle("Numeric"=w229, "String"=w230) -> (→"Progress":cluster{"Numeric":dbl, "String":string})  [unwired: 1 in]
          }
          frame "" {
            n121 = property on="Progress" class="Clust (strict)"("Visible"=FALSE) -> ()  [unwired: 2 in, 2 out]
            n122 = local write "Test Name"(u16 0) -> ()
          }
        }
        n123 = call <vilib>:"Connextion Info.vi"() -> ("Connected"=→"NT Connection":bool)  [unwired: 10 in, 1 out]
      }
      event "Test Tree": Value Change {
        # "Show appropriate\ncontrols"
        n124 = event-data() -> ("CtlRef"=w239:refnum<vi>, "NewVal"=w237:string)  [unwired: 1 in]
        n125 = call <vilib>:"WPI_UtilitiesGetTreeIOName.vi"("NewVal"=w237, "TreeControl in"=w239) -> ("I/O Name"=w240:string)  [unwired: 9 in]
        n126 = case shown="\"Analog Out\", \"Motor\", \"PWM\"" w240 {
          selector: w240 -> [_ w247 _ w269 w278 _]
          tunnel: w237 -> [_ _ w266 w268 _ w285]
          tunnel: w236 -> [_ _ _ _ _ w284]
          frame Default {
            w242 = FALSE ("Visible")
            w241 = FALSE ("Visible")
            n127 = property on="Motor" class="Clust (strict)"("Visible"=w241) -> ()  [unwired: 2 in, 2 out]
            n128 = property on="Test Ring" class="Ring (strict)"("Visible"=w241) -> ()  [unwired: 2 in, 2 out]
            n129 = property on="Rev/Fwd" class="Clust (strict)"("Visible"=w242) -> ()  [unwired: 2 in, 2 out]
            n130 = property on="On/Off" class="Bool (strict)"("Visible"=w242) -> ()  [unwired: 2 in, 2 out]
            n131 = property on="Test Slider" class="Slide (strict)"("Visible"=w242) -> ()  [unwired: 2 in, 2 out]
          }
          frame "Analog Out", "Motor", "PWM" {
            w248 = FALSE ("Visible")
            n132 = case shown="\"Analog Out\"" w247 {
              tunnel: [1.0 ("Value") -1.0 ("Value") 0.0 ("Value")] -> w246
              tunnel: [255.0 ("Value") 1.0 ("Value") 5.0 ("Value")] -> w245
              tunnel: [128.0 ("Value") 0.0 ("Value") 0.0 ("Value")] -> w244
              tunnel: [64.0 ("Value") 0.5 ("Value") 1.0 ("Value")] -> w243
              frame "PWM" {
              }
              frame "Motor", Default {
              }
              frame "Analog Out" {
              }
            }
            n133 = property on="Motor" class="Clust (strict)"("Visible"=TRUE) -> ()  [unwired: 2 in, 2 out]
            n134 = property on="Value" class="Slide (strict)"("Value"=w244, "Scale.Minimum"=w246, "Scale.Maximum"=w245, "Scale.Increment"=w243) -> ()  [unwired: 2 in, 2 out]
            n135 = property on="On/Off" class="Bool (strict)"("Visible"=w248) -> ()  [unwired: 2 in, 2 out]
            n136 = property on="Test Slider" class="Slide (strict)"("Visible"=w248) -> ()  [unwired: 2 in, 2 out]
            n137 = property on="Test Ring" class="Ring (strict)"("Visible"=w248) -> ()  [unwired: 2 in, 2 out]
            n138 = property on="Rev/Fwd" class="Clust (strict)"("Visible"=w248) -> ()  [unwired: 2 in, 2 out]
          }
          frame "Servo" {
            w264 = FALSE ("Visible")
            n139 = call <vilib>:"NT Read Number.vi"("Name"=w266) -> ("Numeric"=w265:dbl)  [unwired: 9 in, 1 out]
            n140 = property on="Test Slider" class="Slide (strict)"("Visible"=TRUE, "Scale.Maximum"=170.0 ("Scale.Range:Maximum")) -> ()  [unwired: 2 in, 2 out]
            n141 = local write "Test Slider"(w265) -> ()
            n142 = property on="Motor" class="Clust (strict)"("Visible"=w264) -> ()  [unwired: 2 in, 2 out]
            n143 = property on="Rev/Fwd" class="Clust (strict)"("Visible"=w264) -> ()  [unwired: 2 in, 2 out]
            n144 = property on="On/Off" class="Bool (strict)"("Visible"=w264) -> ()  [unwired: 2 in, 2 out]
            n145 = property on="Test Ring" class="Ring (strict)"("Visible"=w264) -> ()  [unwired: 2 in, 2 out]
          }
          frame "Relay", "Solenoid" {
            w267 = FALSE ("Visible")
            n146 = property on="Motor" class="Clust (strict)"("Visible"=w267) -> ()  [unwired: 2 in, 2 out]
            n147 = property on="Test Slider" class="Slide (strict)"("Visible"=w267) -> ()  [unwired: 2 in, 2 out]
            n148 = Search and Replace String(input string=w268, search string="/Value  **", replace string="/Direction") -> (result string=w274:string)  [unwired: 5 in, 3 out]
            n149 = property on="Test Ring" class="Ring (strict)"("Visible"=w267) -> ()  [unwired: 2 in, 2 out]
            n150 = call <vilib>:"NT Read String.vi"("Name"=w274) -> ("String"=w272:string)  [unwired: 9 in, 1 out]
            n151 = Equal?(x="Both directions", y=w272) -> (x = y?=w270:bool)
            n152 = Not(x=w270) -> (.not. x?=w271:bool)
            n153 = property on="Rev/Fwd" class="Clust (strict)"("Visible"=w270) -> ()  [unwired: 2 in, 2 out]
            n154 = property on="On/Off" class="Bool (strict)"("Visible"=w271, "Caption.Text"=w269) -> ()  [unwired: 2 in, 2 out]
          }
          frame "Compressor", "Digital Out" {
            w277 = FALSE ("Visible")
            # "Get direction and finish"
            n155 = property on="Motor" class="Clust (strict)"("Visible"=w277) -> ()  [unwired: 2 in, 2 out]
            n156 = property on="Test Slider" class="Slide (strict)"("Visible"=w277) -> ()  [unwired: 2 in, 2 out]
            n157 = property on="Test Ring" class="Ring (strict)"("Visible"=w277) -> ()  [unwired: 2 in, 2 out]
            n158 = property on="On/Off" class="Bool (strict)"("Visible"=TRUE, "Caption.Text"=w278) -> ()  [unwired: 2 in, 2 out]
            n159 = property on="Rev/Fwd" class="Clust (strict)"("Visible"=FALSE) -> ()  [unwired: 2 in, 2 out]
          }
          frame "Camera" {
            n160 = call <vilib>:"Get Last Path Segment.vi"("String in"=w285) -> ("String out"=w286:string)  [unwired: 10 in]
            n161 = property on="On/Off" class="Bool (strict)"("Visible"=FALSE) -> ()  [unwired: 2 in, 2 out]
            n162 = property on="Motor" class="Clust (strict)"("Visible"=FALSE) -> ()  [unwired: 2 in, 2 out]
            n163 = property on="Rev/Fwd" class="Clust (strict)"("Visible"=FALSE) -> ()  [unwired: 2 in, 2 out]
            n164 = case shown="\"White Balance  **\"" w286 {
              tunnel: w285 -> [w292 w301 w310 w319 w328 _ w334]
              tunnel: w284 -> [w290 w298 w307 w316 w325 _ _]
              frame "Size  **" {
                n165 = Index Array(array=w290) -> (element=w289:cluster{string[]})  [unwired: 1 in]
                n166 = call <vilib>:"NT Read String.vi"("Name"=w292) -> ("String"=w291:string)  [unwired: 9 in, 1 out]
                n167 = Unbundle(w289) -> (w287:string[])
                n168 = Match First String(2:w287, 3:w291) -> (0:w288:i32)  [unwired: 1 out]
                n169 = property on="Test Ring" class="Ring (strict)"("Value"=w288, "Strings []"=w287) -> ()  [unwired: 2 in, 2 out]
                n170 = property on="Test Ring" class="Ring (strict)"("Visible"=TRUE) -> ()  [unwired: 2 in, 2 out]
                n171 = property on="Test Slider" class="Slide (strict)"("Visible"=FALSE) -> ()  [unwired: 2 in, 2 out]
              }
              frame "White Balance  **" {
                n172 = Index Array(array=w298, index=1) -> (element=w299:cluster{string[]})
                n173 = call <vilib>:"NT Read String.vi"("Name"=w301) -> ("String"=w300:string)  [unwired: 9 in, 1 out]
                n174 = Unbundle(w299) -> (w296:string[])
                n175 = Match First String(2:w296, 3:w300) -> (0:w295:i32)  [unwired: 1 out]
                n176 = property on="Test Ring" class="Ring (strict)"("Value"=w295, "Strings []"=w296) -> ()  [unwired: 2 in, 2 out]
                n177 = property on="Test Ring" class="Ring (strict)"("Visible"=TRUE) -> ()  [unwired: 2 in, 2 out]
                n178 = property on="Test Slider" class="Slide (strict)"("Visible"=FALSE) -> ()  [unwired: 2 in, 2 out]
              }
              frame "Exposure  **" {
                n179 = Index Array(array=w307, index=2) -> (element=w308:cluster{string[]})
                n180 = call <vilib>:"NT Read String.vi"("Name"=w310) -> ("String"=w309:string)  [unwired: 9 in, 1 out]
                n181 = Unbundle(w308) -> (w304:string[])
                n182 = Match First String(2:w304, 3:w309) -> (0:w305:i32)  [unwired: 1 out]
                n183 = property on="Test Ring" class="Ring (strict)"("Value"=w305, "Strings []"=w304) -> ()  [unwired: 2 in, 2 out]
                n184 = property on="Test Ring" class="Ring (strict)"("Visible"=TRUE) -> ()  [unwired: 2 in, 2 out]
                n185 = property on="Test Slider" class="Slide (strict)"("Visible"=FALSE) -> ()  [unwired: 2 in, 2 out]
              }
              frame "Exposure Priority  **" {
                n186 = Index Array(array=w316, index=3) -> (element=w317:cluster{string[]})
                n187 = call <vilib>:"NT Read String.vi"("Name"=w319) -> ("String"=w318:string)  [unwired: 9 in, 1 out]
                n188 = Unbundle(w317) -> (w313:string[])
                n189 = Match First String(2:w313, 3:w318) -> (0:w314:i32)  [unwired: 1 out]
                n190 = property on="Test Ring" class="Ring (strict)"("Value"=w314, "Strings []"=w313) -> ()  [unwired: 2 in, 2 out]
                n191 = property on="Test Ring" class="Ring (strict)"("Visible"=TRUE) -> ()  [unwired: 2 in, 2 out]
                n192 = property on="Test Slider" class="Slide (strict)"("Visible"=FALSE) -> ()  [unwired: 2 in, 2 out]
              }
              frame "Color Enable  **" {
                n193 = Index Array(array=w325, index=4) -> (element=w326:cluster{string[]})
                n194 = call <vilib>:"NT Read String.vi"("Name"=w328) -> ("String"=w327:string)  [unwired: 9 in, 1 out]
                n195 = Unbundle(w326) -> (w322:string[])
                n196 = Match First String(2:w322, 3:w327) -> (0:w323:i32)  [unwired: 1 out]
                n197 = property on="Test Ring" class="Ring (strict)"("Value"=w323, "Strings []"=w322) -> ()  [unwired: 2 in, 2 out]
                n198 = property on="Test Ring" class="Ring (strict)"("Visible"=TRUE) -> ()  [unwired: 2 in, 2 out]
                n199 = property on="Test Slider" class="Slide (strict)"("Visible"=FALSE) -> ()  [unwired: 2 in, 2 out]
              }
              frame Default {
                n200 = property on="Test Ring" class="Ring (strict)"("Visible"=FALSE) -> ()  [unwired: 2 in, 2 out]
                n201 = property on="Test Slider" class="Slide (strict)"("Visible"=FALSE) -> ()  [unwired: 2 in, 2 out]
              }
              frame "Brightness  **", "Color Level  **", "Compression  **", "FPS  **", "Sharpness  **" {
                n202 = call <vilib>:"NT Read Number.vi"("Name"=w334) -> ("Numeric"=w333:dbl)  [unwired: 9 in, 1 out]
                n203 = local write "Test Slider"(w333) -> ()
                n204 = property on="Test Slider" class="Slide (strict)"("Visible"=TRUE, "Scale.Maximum"=100.0 ("Scale.Range:Maximum")) -> ()  [unwired: 2 in, 2 out]
                n205 = property on="Test Ring" class="Ring (strict)"("Visible"=FALSE) -> ()  [unwired: 2 in, 2 out]
              }
            }
          }
        }
        n206 = property on="Progress" class="Clust (strict)"("Visible"=FALSE) -> ()  [unwired: 2 in, 2 out]
      }
      event "Test Name": Mouse Enter {
        # "Populate the ring with the list of tests"
        n207 = event-data() -> ()  [unwired: 1 in, 1 out]
        n208 = call <vilib>:"NT Read String Array.vi"("Name"="/TestMode/TestList") -> ("String Array"=w343:string[])  [unwired: 9 in, 1 out]
        n209 = Build Array (concatenate)("Select the test to run...", w343) -> (w342:string[])
        n210 = property on="Test Name" class="Ring (strict)"("Strings []"=w342) -> ()  [unwired: 2 in, 2 out]
      }
      event "Test Name": Value Change {
        w346 = FALSE ("Visible")
        # "Tell the robot the test name to run"
        n211 = event-data() -> ("NewVal"=w350:u16)  [unwired: 1 in]
        n212 = property on="Test Name" class="Ring (strict)"() -> ("Strings []"=w351:string[])  [unwired: 2 in, 2 out]
        n213 = local write "Progress"(T7 {"Test Progress"=0, "Test Progress Text"=""} ("Progress")) -> ()
        n214 = Index Array(array=w351, index=w350) -> (element=w349:string)
        n215 = call <vilib>:"NT Write String.vi"("String"=w349, "Name"="/TestMode/TestName") -> ()  [unwired: 9 in, 1 out]
        n216 = property on="Progress" class="Clust (strict)"("Visible"=TRUE) -> ()  [unwired: 2 in, 2 out]
        n217 = property on="Motor" class="Clust (strict)"("Visible"=w346) -> ()  [unwired: 2 in, 2 out]
        n218 = property on="Test Slider" class="Slide (strict)"("Visible"=w346) -> ()  [unwired: 2 in, 2 out]
        n219 = property on="On/Off" class="Bool (strict)"("Visible"=w346) -> ()  [unwired: 2 in, 2 out]
        n220 = property on="Rev/Fwd" class="Clust (strict)"("Visible"=w346) -> ()  [unwired: 2 in, 2 out]
        n221 = property on="Test Ring" class="Ring (strict)"("Visible"=w346) -> ()  [unwired: 2 in, 2 out]
      }
      event "Select Auto": Mouse Enter {
        # "Populate the combo box with the list of autonomous options"
        n222 = event-data() -> ()  [unwired: 1 in, 1 out]
        n223 = call <vilib>:"NT Read String Array.vi"("Name"="Auto List") -> ("String Array"=w353:string[])  [unwired: 9 in, 1 out]
        n224 = property on="Select Auto" class="CmbBox"("Strings[]"=w353) -> ()  [unwired: 2 in, 2 out]
      }
      event "Select Auto": Value Change {
        # "User modified the Auto Selection. Write to NT variable so robot knows."
        n225 = event-data() -> ("NewVal"=w357:string)  [unwired: 1 in]
        n226 = call <vilib>:"NT Write String.vi"("String"=w357, "Name"="Auto Selector") -> ()  [unwired: 9 in, 1 out]
      }
      event "Command Selection": Value Change {
        # "Get the params and show in table"
        n227 = event-data() -> ("NewVal"=w364:i32)  [unwired: 1 in]
        n228 = property on="Command Selection" class="MCListbox (strict)"() -> ("ItemNames"=w362:string[][])  [unwired: 2 in, 2 out]
        n229 = call <vilib>:"WPI_DashboardUpdate Command Params.vi"("NewVal"=w364, "Commands"=w362, "Param Tbl"=w363) -> ()  [unwired: 8 in, 1 out]
      }
      event "Execute Command": Value Change {
        # "Started one, Unique ID holds\nresponse"
        n230 = event-data() -> ()  [unwired: 1 in, 1 out]
        n231 = property on="Command Selection" class="MCListbox (strict)"() -> ("ItemNames"=w376:string[][])  [unwired: 2 in, 2 out]
        n232 = Index Array(array=w376, index (row)="Command Selection", index (col)=0) -> (element=w374:string)
        n233 = call <vilib>:"Invoke Commands.vi"("Command Params"="Command Params", "Function Name"=w374) -> ("Params"=w370:u8, "Started"=w369:bool)  [unwired: 7 in, 1 out]
        n234 = Array Subset(array="Command Params", length (row)=w370) -> (w371:string[][])  [unwired: 3 in]
        n235 = Select(t="Executing" ("Cmd Status"), s=w369, f="" ("Cmd Status")) -> (s? t:f=→"Cmd Status":string)
      }
      event "Command Selection": Double Click {
        n236 = event-data() -> ("Row"=w386:i32)  [unwired: 1 in]
        n237 = property on="Command Selection" class="MCListbox (strict)"() -> ("ItemNames"=w389:string[][])  [unwired: 2 in, 2 out]
        n238 = local read "Command Params"() -> (w384:string[][])
        n239 = Index Array(array=w389, index (row)=w386, index (col)=0) -> (element=w387:string)
        n240 = call <vilib>:"Invoke Commands.vi"("Command Params"=w384, "Function Name"=w387) -> ("Params"=w383:u8, "Started"=w378:bool)  [unwired: 7 in, 1 out]
        n241 = Array Subset(array=w384, length (row)=w383) -> (w382:string[][])  [unwired: 3 in]
        n242 = Select(t="Executing" ("Cmd Status"), s=w378, f="" ("Cmd Status")) -> (s? t:f=w379:string)
        n243 = local write "Cmd Status"(w379) -> ()
      }
      event "CheckList": Double Click {
        # "Shift clears all"
        # "Update symbols on the listbox"
        n244 = event-data() -> ("PlatMods.Shift"=w392:bool, "Row"=w394:i32)  [unwired: 1 in]
        n245 = case shown="True" w392 {
          tunnel: w394 -> [w398 _]
          tunnel: 1 -> [w397 _]
          frame False {
            n246 = property on="CheckList" class="LstBox (strict)"() -> ("Item Symbols"=w396:i32[])  [unwired: 2 in, 2 out]
            n247 = Replace Array Subset(array=w396, new element=w397, index=w398) -> (w395:i32[])
            n248 = property on="CheckList" class="LstBox (strict)"("Item Symbols"=w395) -> ()  [unwired: 2 in, 2 out]
          }
          frame True {
            w399 = 0 ("Top Row")
            n249 = property on="CheckList" class="LstBox (strict)"() -> ("Number of Rows"=w401:u32)  [unwired: 2 in, 2 out]
            n250 = Initialize Array(0, w401) -> (w400:i32[])
            n251 = property on="CheckList" class="LstBox (strict)"("Top Row"=w399, "Value"=w399, "Item Symbols"=w400) -> ()  [unwired: 2 in, 2 out]
          }
        }
      }
      event "CheckList": Key Down {
        # "Update symbols on the listbox\nLeft and right keys check and uncheck"
        n252 = event-data() -> ("VKey"=w406:T22)  [unwired: 1 in]
        n253 = case shown="\"Left\", \"Right\"" w406 {
          selector: w406 -> [w411 _]
          tunnel: eventvkey."Left" ("VKey") -> [w409 _]
          frame "Left", "Right" {
            n254 = Equal?(x=w409, y=w411) -> (x = y?=w410:bool)
            n255 = Select(t=0, s=w410, f=1) -> (s? t:f=w412:i32)
            n256 = property on="CheckList" class="LstBox (strict)"() -> ("Item Symbols"=w415:i32[])  [unwired: 2 in, 2 out]
            n257 = Replace Array Subset(array=w415, new element=w412, index="CheckList") -> (w414:i32[])
            n258 = property on="CheckList" class="LstBox (strict)"("Item Symbols"=w414) -> ()  [unwired: 2 in, 2 out]
          }
          frame Default {
          }
        }
      }
      event "DB Camera Config": Value Change {
        # "Show or hide the cluster of controls, store in ini file"
        n259 = event-data() -> ("NewVal"=w420:bool)  [unwired: 1 in]
        n260 = case shown="False" w420 {
          tunnel: w419 -> [w429 _]
          tunnel: [w422 w440] -> w418
          tunnel: w417 -> [w421 w440]
          frame False {
            w436 = "Camera"
            w439 = FALSE ("Visible")
            n261 = local read "Camera Settings"() -> (w428:T2)
            n262 = Index Array(array=w429) -> (element=w432:cluster{string[]})  [unwired: 1 in]
            n263 = Unbundle(w428) -> ("Frame Rate"=w427:i32, "Compression"=w426:i32, "Size"=w430:u16)
            n264 = Unbundle(w432) -> (w431:string[])
            n265 = Index Array(array=w431, index=w430) -> (element=w425:string)
            n266 = call-poly <vilib>:"Write Key.vi"("section"=w436, "value"=w425, "key"="Size", "refnum"=w421) -> ("refnum out"=w438:T20)  [unwired: 2 in, 5 out]
            n267 = call-poly <vilib>:"Write Key.vi"("section"=w436, "value"=w427, "key"="FrameRate", "refnum"=w438) -> ("refnum out"=w437:T20)  [unwired: 1 in, 6 out]
            n268 = property on="Camera Settings" class="Clust (strict)"("Visible"=w439) -> ()  [unwired: 2 in, 2 out]
            n269 = local write "DB Camera Config"(w439) -> ()
            n270 = call-poly <vilib>:"Write Key.vi"("section"=w436, "value"=w426, "key"="Compression", "refnum"=w437) -> ("refnum out"=w423:T20)  [unwired: 1 in, 6 out]
            n271 = call <vilib>:"Close Config Data.vi"("refnum"=w423) -> ("file path"=w424:path)  [unwired: 2 in, 8 out]
            n272 = call <vilib>:"Open Config Data.vi"("configuration file path"=w424) -> ("refnum"=w422:T20)  [unwired: 8 in, 2 out]
          }
          frame True {
            n273 = property on="Camera Settings" class="Clust (strict)"("Visible"=TRUE) -> ()  [unwired: 2 in, 2 out]
          }
        }
      }
      event "Camera Settings": Value Change {
        # "Update summary string when any elements of DB camera change"
        n274 = event-data() -> ("NewVal"=w454:T2)  [unwired: 1 in]
        n275 = Index Array(array=w450) -> (element=w449:cluster{string[]})  [unwired: 1 in]
        n276 = Unbundle(w454) -> ("Frame Rate"=w445:i32, "Compression"=w444:i32, "Size"=w447:u16)
        n277 = Unbundle(w449) -> (w448:string[])
        n278 = Index Array(array=w448, index=w447) -> (element=w446:string)
        n279 = Format Into String(format string="%s   %dfps   %d%%", w446, w445, w444) -> (resulting string=w451:string)  [unwired: 2 in, 1 out]
        n280 = Build Array(w451) -> (w452:string[])
        n281 = property on="DB Camera Config" class="Bool (strict)"("Strings [4]"=w452) -> ()  [unwired: 2 in, 2 out]
      }
      event "Motor.Enable": Value Change {
        # "When the test mode otor enable helper is set, update that\ntree row item's value"
        n282 = event-data() -> ("NewVal"=w461:bool)  [unwired: 1 in]
        n283 = Unbundle("Motor") -> ("Value"=w460:dbl)  [unwired: 1 out]
        n284 = Select(t=w460, s=w461, f=0.0) -> (s? t:f=w458:dbl)
        n285 = call <vilib>:"NT Write Number.vi"("Numeric"=w458, "Name"=w457) -> ()  [unwired: 9 in, 1 out]
      }
      event "Test Slider": Value Change {
        # "When the test mode slider helper is set, update that\ntree row item's value"
        n286 = event-data() -> ("NewVal"=w465:dbl)  [unwired: 1 in]
        n287 = call <vilib>:"NT Write Number.vi"("Numeric"=w465, "Name"=w466) -> ()  [unwired: 9 in, 1 out]
      }
      event "On/Off": Value Change {
        # "When the test mode on/off helper value is set, update that\ntree row item's value"
        n288 = event-data() -> ("NewVal"=w471:bool)  [unwired: 1 in]
        n289 = Boolean To (0,1)(Boolean=w471) -> (0, 1=w470:i16)
        n290 = call <vilib>:"NT Write Number.vi"("Numeric"=w470, "Name"=w469) -> ()  [unwired: 9 in, 1 out]
      }
      event "Rev/Fwd": Value Change {
        # "When the test mode helper value for relays is set, update that\ntree row item's value"
        n291 = event-data() -> ("NewVal.Forward"=w480:bool, "NewVal.Reverse"=w479:bool)  [unwired: 1 in]
        n292 = Boolean To (0,1)(Boolean=w480) -> (0, 1=w476:i16)
        n293 = Boolean To (0,1)(Boolean=w479) -> (0, 1=w478:i16)
        n294 = Negate(x=w478) -> (-x=w477:i16)
        n295 = Add(x=w476, y=w477) -> (x+y=w475:i16)
        n296 = call <vilib>:"NT Write Number.vi"("Numeric"=w475, "Name"=w474) -> ()  [unwired: 9 in, 1 out]
      }
      event "Test Ring": Value Change {
        # "When a test mode helper value is selected from the ring,\nset the tree item's variable to the string value"
        n297 = event-data() -> ("NewVal"=w485:u16)  [unwired: 1 in]
        n298 = property on="Test Ring" class="Ring (strict)"() -> ("Strings []"=w486:string[])  [unwired: 2 in, 2 out]
        n299 = Index Array(array=w486, index=w485) -> (element=w484:string)
        n300 = call <vilib>:"NT Write String.vi"("String"=w484, "Name"=w483) -> ()  [unwired: 9 in, 1 out]
      }
      event "Rec Mode": Value Change {
        # "Update globals for recording mode and path to read log from.\nClear when logging and let NetworkTables set path for vision to\nuse."
        n301 = event-data() -> ("NewVal"=w498:enum32{"Stop", "Record", "Playback"})  [unwired: 1 in]
        n302 = global write "WPI_DashboardLogging Global.vi" "Logging Filename"(path "") -> ()
        n303 = global write "WPI_DashboardLogging Global.vi" "Recording"(w498) -> ()
        n304 = case shown="\"Playback\"" w498 {
          tunnel: w497 -> [_ w500 w509]
          tunnel: [_ _ w508] -> w494
          tunnel: [_ _ w507] -> _
          tunnel: w492 -> [_ _ w505]
          tunnel: cluster{i32, i32} {-250, 170} -> [_ _ w504]
          tunnel: [_ _ T23 {"Image Size"=TRUE, "Image Type"=TRUE, "Pixel Value"=TRUE, "ROI Information"=TRUE, "Zoom Factor"=FALSE} ("Image Information Shown:All Elements")] -> w490
          tunnel: [_ _ TRUE ("Zoom Factor")] -> w489
          tunnel: w488 -> [_ _ w501]
          frame Default {
          }
          frame "Stop", "Record" {
            # "Place Window too"
            n305 = invoke class="VI" method="FP.Close"(reference=w500) -> (reference out=w499:refnum<vi>)  [unwired: 2 in, 2 out]
            n306 = invoke class="VI" method="Abort VI"(reference=w499) -> ()  [unwired: 2 in, 3 out]
          }
          frame "Playback" {
            n307 = call "Open Playback Panel.vi"("Offset"=w504, "DB VI Ref"=w505, "Playback in"=w509) -> ("Playback out"=w506:refnum<vi>)  [unwired: 8 in]
            n308 = register-events(w506, w501) -> (reference out=w508:refnum<event-registration>, error out=w507:errorcluster)  [unwired: 2 in]
          }
        }
        n309 = property on="Camera Image" class="ImageControl"("Image Information Shown"=w490, "Image Information Visible"=w489) -> ()  [unwired: 2 in, 2 out]
        n310 = call <vilib>:"WPI_DashboardNT Log FieldName Cache.vi"("Operation"=enum16{"Lookup/Add", "Index", "Clear"}."Clear") -> ()  [unwired: 8 in, 3 out]
      }
      event Panel Close {
        w511 = enum32{"Stop", "Record", "Playback"}."Stop" ("Rec Mode")
        # "Playback window has been closed, abort"
        n311 = event-data() -> ()  [unwired: 1 in, 4 out]
        n312 = local write "Rec Mode"(w511) -> ()
        n313 = global write "WPI_DashboardLogging Global.vi" "Recording"(w511) -> ()
      }
      event Panel Close {
        # "Abort playback window and ourself"
        n314 = event-data() -> ()  [unwired: 1 in, 4 out]
        n315 = invoke class="VI" method="FP.Close"(reference=w517) -> (reference out=w516:refnum<vi>)  [unwired: 2 in, 2 out]
        n316 = invoke class="VI" method="Abort VI"(reference=w516) -> (error out=w515:errorcluster)  [unwired: 2 in, 2 out]
        n317 = invoke class="VI" method="Abort VI"(error in=w515) -> ()  [unwired: 2 in, 3 out]
      }
      event User Event {
        n318 = event-data() -> ("IDs"=w525:cluster{"RPC field ID":u16, "Unique ID":u16}, "String"=w524:string)  [unwired: 1 in]
        n319 = Bundle("IDs"=w525, "String"=w524) -> (w523:T9)  [unwired: 1 in]
        n320 = call <vilib>:"Retrieve RPC Response.vi"("RPC Response"=w523) -> ("Output"=w520:string[][])  [unwired: 10 in]
        n321 = Build Array (concatenate)(w518, w520) -> (w519:string[][])
        n322 = local write "Command Params"(w519) -> ()
        n323 = local write "Cmd Status"("" ("Cmd Status")) -> ()
      }
      event "Vision": Value Change {
        # "Enable/Disable Compression slider.\nHW USB is hard-coded into the camera"
        n324 = event-data() -> ("NewVal"=w532:u16)  [unwired: 1 in]
        n325 = Equal?(x=w532, y=u32 2 ("milliseconds to wait")) -> (x = y?=w530:bool)
        n326 = Select(t=T24."Disabled and Grayed Out" ("Disabled"), s=w530, f=T24."Enabled" ("Disabled")) -> (s? t:f=w527:T24)
        n327 = property on="Compression" class="Slide (strict)"("DisabledEnum"=w527) -> ()  [unwired: 2 in, 2 out]
      }
      event "Tree": Double Click {
        n328 = event-data() -> ("PlatMods"=w537:T27, "Tag"=w536:string)  [unwired: 1 in]
        n329 = Unbundle(w537) -> ("Shift"=w535:bool)  [unwired: 4 out]
        n330 = Not(x=w535) -> (.not. x?=w534:bool)
        n331 = call <vilib>:"NT Update Persistence.vi"("Persistence"=w534, "Name"=w536) -> ()  [unwired: 9 in, 1 out]
      }
    }
  }
  n332 = while {
    tunnel: w47 -> [w541]
    i -> [w544]
    stop <- FALSE stop-if-true
    n333 = Wait (ms)(milliseconds to wait=u32 100) -> ()  [unwired: 1 out]
    n334 = case shown="\"Playback\"" "Rec Mode" {
      tunnel: w544 -> [_ _ w559]
      tunnel: [u32 2829099 ("Base Color") u32 11141120 ("Target Color") w548] -> w540
      frame "Stop", Default {
        # "Reset the color, extra updates don't cost much"
      }
      frame "Record" {
      }
      frame "Playback" {
        # "Playback"
        n335 = Quotient & Remainder(x=w559, y=u32 50 ("milliseconds to wait")) -> (x-y*floor(x/y)=w555:u32)  [unwired: 1 out]
        n336 = Divide(x=w555, y=u32 50 ("milliseconds to wait")) -> (x/y=w552:dbl)
        n337 = Multiply(x=6.283185307179586, y=w552) -> (x*y=w557:dbl)
        n338 = Sine(x=w557) -> (sin(x)=w556:dbl)
        n339 = Absolute Value(x=w556) -> (abs(x)=w549:dbl)
        n340 = call "Interpolate RGB Color.vi"("Proportion"=w549, "Target Color"=u32 30976, "Base Color"=u32 2829099) -> ("Result Color"=w548:u32)  [unwired: 8 in]
      }
    }
    n341 = property class="Pane"(reference=w541, "PaneColor"=w540) -> ()  [unwired: 1 in, 2 out]
  }
  n342 = local write "Dashboard Tab"(T1."Drive" ("Dashboard Tab")) -> ()
  n343 = property on="On/Off" class="Bool (strict)"("Visible"=w15) -> ()  [unwired: 2 in, 2 out]
  n344 = property on="Motor" class="Clust (strict)"("Visible"=w15) -> ()  [unwired: 2 in, 2 out]
  n345 = property on="Progress" class="Clust (strict)"("Visible"=w15) -> ()  [unwired: 2 in, 2 out]
  n346 = property on="Test Ring" class="Ring (strict)"("Visible"=w15) -> ()  [unwired: 2 in, 2 out]
  n347 = property on="Rev/Fwd" class="Clust (strict)"("Visible"=w15) -> ()  [unwired: 2 in, 2 out]
  n348 = property on="Camera Settings" class="Clust (strict)"("Visible"=w15) -> ()  [unwired: 2 in, 2 out]
  n349 = local write "DB Camera Config"(w15) -> ()
  n350 = while {
    tunnel: u16 1741 ("timeout ms (25000)") -> [w561]
    stop <- FALSE stop-if-true
    n351 = TCP Create Listener(10:w561) -> (0:w560:errorcluster, 3:w562:refnum<k5>)  [unwired: 4 in, 1 out]
    n352 = case shown="No Error" w560 {
      selector: w560 -> [w564 _]
      tunnel: w562 -> [w565 _]
      frame No Error {
        n353 = while {
          tunnel: w565 -> [w568]
          tunnel: w564 -> [w567]
          stop <- FALSE stop-if-true
          n354 = TCP Wait On Listener(8:w567, 11:w568) -> (0:w569:errorcluster, 4:w570:refnum<k5>)  [unwired: 2 in, 3 out]
          n355 = local write "TCP"(w570) -> ()
          n356 = case shown="No Error" w569 {
            frame No Error {
            }
            frame Error {
              n357 = Wait (ms)(milliseconds to wait=u32 1000) -> ()  [unwired: 1 out]
            }
          }
        }
      }
      frame Error {
        n358 = Wait (ms)(milliseconds to wait=u32 1000) -> ()  [unwired: 1 out]
      }
    }
  }
  n359 = local write "Command Params"(string[][] [] ("Command Params")) -> ()
  n360 = global write "WPI_DashboardLogging Global.vi" "Recording"(w41) -> ()
  n361 = local write "Rec Mode"(w41) -> ()
  n362 = local write "Command Selection"(u16 0 ("milliseconds to wait")) -> ()
